vi "Move Replicate Sq1.vi"(10 "View":i32[](array[numeric]) caption="View (Team Index, -1: empty)") -> (1 "Direction":T2, 2 "Action":T1)   [LabVIEW 2015, in "AndrewF.lvclass"]
uses:
  AndrewF.lvclass
  Type Defs/Direction Enum.ctl
  Type Defs/Action Enum.ctl
  Type Defs/SB Type Defs.lvlib
  Common/Common.lvlib
panel:
  # "NW\nN\nNE\nE\nSE\nS\nSW\nW"
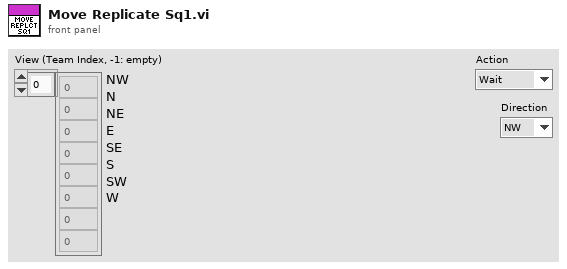
[diagram p1: front panel]
types:
  T1 = typedef "SB Type Defs.lvlib/Action Enum.ctl" = enum16{"Wait", "Move", "Attack", "Replicate"}
  T2 = typedef "SB Type Defs.lvlib/Direction Enum.ctl" = enum16{"NW", "N", "NE", "E", "SE", "S", "SW", "W"}
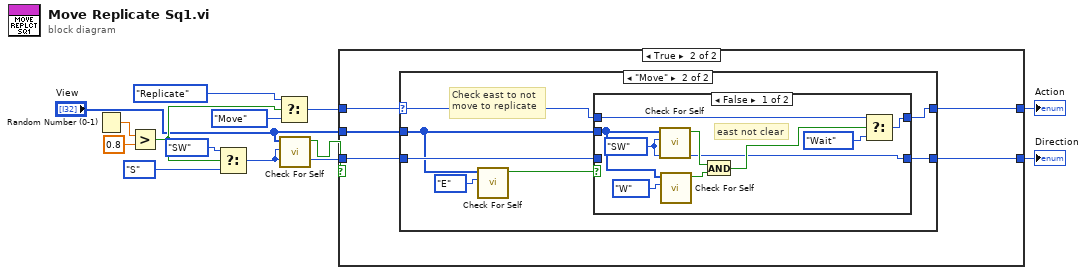
[diagram p0: block diagram]
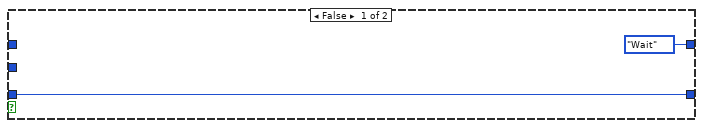
[diagram p2: hidden frame]
diagram:
  n1 = Random Number (0-1)() -> (number: 0 to 1=w13:dbl)
  n2 = Greater?(x=w13, y=0.8) -> (0:w7:bool)
  n3 = Select(t=Direction_Enum."SW" ("Direction"), s=w7, f=Direction_Enum."S") -> (s? t:f=w3:T2)
  n4 = Select(t=Action_Enum."Replicate" ("Action"), s=w7, f=Action_Enum."Move" ("Action")) -> (s? t:f=w4:T1)
  n5 = call "Check For Self.vi"("Direction"=w3, "Map"="View") -> ("Clear?"=w5:bool)  [unwired: 9 in]
  n6 = case shown="True" w5 {
    tunnel: "View" -> [_ w20]
    tunnel: w4 -> [_ w18]
    tunnel: [w14 w16] -> w2
    tunnel: w3 -> [w14 w17]
    tunnel: [Action_Enum."Wait" ("f") w19] -> w1
    frame False {
    }
    frame True {
      n7 = case shown="\"Move\"" w18 {
        selector: w18 -> [w22 w26]
        tunnel: w20 -> [_ w24]
        tunnel: [w22 w25] -> w19
        tunnel: w17 -> [w21 w28]
        tunnel: [w21 w27] -> w16
        frame "Wait", Default {
        }
        frame "Move" {
          # "Check east to not\nmove to replicate"
          n8 = call "Check For Self.vi"("Direction"=Direction_Enum."E", "Map"=w24) -> ("Clear?"=w23:bool)  [unwired: 9 in]
          n9 = case shown="False" w23 {
            tunnel: w28 -> [_ w39]
            tunnel: [w30 w39] -> w27
            tunnel: w26 -> [w38 w40]
            tunnel: [w36 w40] -> w25
            tunnel: w24 -> [w34 _]
            frame False {
              w30 = Direction_Enum."SW" ("Direction")
              # "east not clear"
              n10 = call "Check For Self.vi"("Direction"=w30, "Map"=w34) -> ("Clear?"=w33:bool)  [unwired: 9 in]
              n11 = call "Check For Self.vi"("Direction"=Direction_Enum."W", "Map"=w34) -> ("Clear?"=w32:bool)  [unwired: 9 in]
              n12 = And(x=w33, y=w32) -> (x .and. y?=w31:bool)
              n13 = Select(t=w38, s=w31, f=Action_Enum."Wait") -> (s? t:f=w36:T1)
            }
            frame True {
            }
          }
        }
      }
    }
  }
  "Direction" <- w2
  "Action" <- w1
